vi "OpenALPR_Init.vi"(8 "error in (no error)":errorcluster, 10 "Max possibility":i32=3, 11 "Default Country":string="hu") -> (0 "error out":errorcluster, 3 "Error":string)   [LabVIEW 2014, in "OpenALPR in LabView.lvlib"]
doc: "Initialize the OpenALPR library.\n\n!!! YOU HAVE TO HAVE A \"OPENALPR_PATH\" ENVIRONMENT VARIABLE WITH THE \"openalpr_32\" DIRECTORY WITCH CONTAINS THE CONFIG FILE AND THE RUNTIME DIRECTORY TO THE SUCCELFUL LOAD! !!!\n\nextern \"C\" __declspec(dllexport) char* OALPRLabVIEW_Init(char* defReg, int topN);"
uses:
  OpenALPR in LabView.lvlib
  Dlls/OALPRLabVIEW.dll
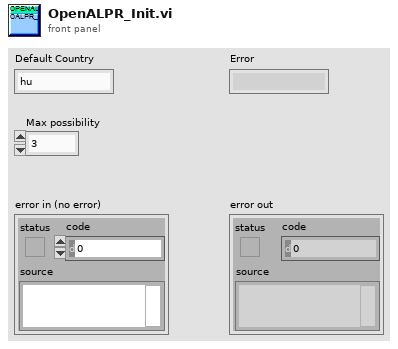
[diagram p1: front panel]
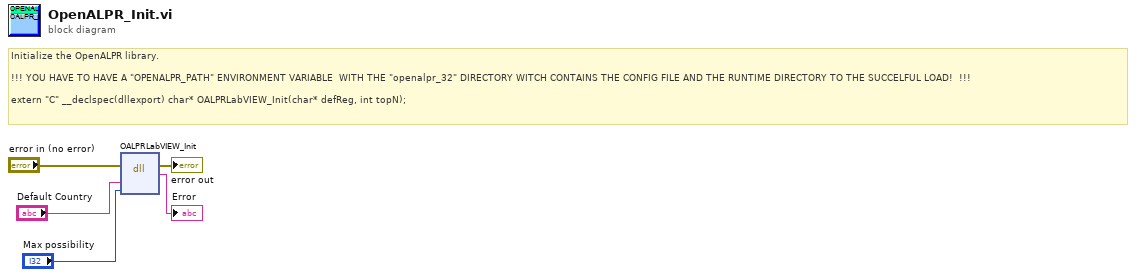
[diagram p0: block diagram]
diagram:
  # "Initialize the OpenALPR library.\n\n!!! YOU HAVE TO HAVE A \"OPENALPR_PATH\" ENVIRONMENT VARIABLE  WITH THE \"openalpr_32\" DIRECTORY WITCH CONTAINS THE CONFIG FILE AND THE RUNTIME DIRECTORY TO THE SUCCELFUL LOAD!  !!!\n\nextern \"C\" __declspec(dllexport) char* OALPRLabVIEW_Init(char* defReg, int topN);"
  n1 = dll-call lib="PTH2abs EFelhasznÃ¡lÃ³kPixelbetyÃ¡rDesktopC19 -C3 Verseny bekÃ¼ldÃ©shez\tSmartMarkOpenALPR to LVOpenALPR_LabVIEWDllsOALPRLabVIEW.*" fn="OALPRLabVIEW_Init"(error in="error in (no error)", "Default Country"="Default Country", "Max possibility"="Max possibility") -> (error out=→"error out":errorcluster, "return type"=→"Error":string)  [unwired: 4 in, 1 out]
